vi "MotionCapture0429.vi"() -> ()   [LabVIEW 2020]
uses:
  <vilib>/Math Plots/3D Math Plots/3D Scatter/3D Scatter XCtrl/3D Scatter.xctl
  <vilib>/Math Plots/3D Math Plots/3D Scatter/3D Scatter Datatype/3D Scatter Datatype.lvclass
  <vilib>/imath/engines/lvmath2/RunTimeEngine/IndexRead/NIMS V(S).vi
  <instcachedir>/0/NIMS V(S)_0488751826AF41519A22953C041130DC.lvgen/NIMS V(S)_0488751826AF41519A22953C041130DC_000.vi
  <vilib>/imathl/engines/lvmath/Functions/Error Handling/Create Error.vi
  <vilib>/imath/engines/lvmath2/RunTimeEngine/BuiltInFunctions/norm/NIMS_norm(GV,DBL).vi
  <instcachedir>/0/NIMS_norm(GV,DBL)_118B4CCB667A4D7498CD7C123070720C.lvgen/NIMS_norm(GV,DBL)_118B4CCB667A4D7498CD7C123070720C_000.vi
  <vilib>/imath/engines/lvmath2/RunTimeEngine/BuiltInFunctions/dot/NIMS_dot(GV,GV).vi
  <instcachedir>/0/NIMS_dot(GV,GV)_B9FAA411F4494E9B94D442721014A3FA.lvgen/NIMS_dot(GV,GV)_B9FAA411F4494E9B94D442721014A3FA_000.vi
  <vilib>/imath/engines/lvmath2/RunTimeEngine/ErrorHandling/NIMS_Create Error From Enums.vi
  <vilib>/imath/engines/lvmath2/RunTimeEngine/BuiltInFunctions/atan2/NIMS_atan2.vi
  <instcachedir>/0/NIMS_atan2_A91AA4A7D42247EDBE8F76DB99AF04A4.lvgen/NIMS_atan2_A91AA4A7D42247EDBE8F76DB99AF04A4_000.vi
  <vilib>/imath/engines/lvmath2/RunTimeEngine/BuiltInFunctions/sin/NIMS_sin(C).vi
  <instcachedir>/0/NIMS_sin(C)_5976CC71585441B3B5B50155927B54AC.lvgen/NIMS_sin(C)_5976CC71585441B3B5B50155927B54AC_001.vi
  <vilib>/imath/engines/lvmath2/RunTimeEngine/NodeEndStatement/NIMS_NodeEndStatement_Output.vi
  <instcachedir>/0/NIMS_NodeEndStatement_Output_53EC0D466D134D7ABD903AC30B43404B.lvgen/NIMS_NodeEndStatement_Output_53EC0D466D134D7ABD903AC30B43404B_001.vi
  <instcachedir>/0/NIMS_NodeEndStatement_Output_53EC0D466D134D7ABD903AC30B43404B.lvgen/NIMS_NodeEndStatement_Output_53EC0D466D134D7ABD903AC30B43404B_009.vi
  <vilib>/imath/engines/lvmath2/RunTimeEngine/ErrorHandling/NIMS_Finalize Error.vi
  <vilib>/Math Plots/3D Math Plots/3D Scatter/3D Scatter Datatype/Public/Plot Helper (Vector).vi
panel:
  out "3D Scatter":refnum<class "3D Plot Datatype.lvclass">[](xcontrol) caption="Endpoint Trajectory"
  in  "采集开关":bool=TRUE
  in  "BodyID":dbl=14.0
  out "CMTrackData":T1={"BodyID"=5, "timecode"=1444098, "T"=[230.07000732421875, 348.40191650390625, -6.298731803894043], [0.322020434693915, 0.3319248787086055, 0.6304688324459874, -0.623408185579892]}
  in  "BodyID 2":dbl=1550.0
  out "CMTrackData 2":T1={"BodyID"=1550, "timecode"=1444098, "T"=[269.41546630859375, 348.2109680175781, 32.023807525634766], [0.0, 1.0, 0.0, 0.0]}
  in  "BodyID 3":dbl=1551.0
  out "CMTrackData 3":T1={"BodyID"=1551, "timecode"=1376028, "T"=[269.479248046875, 346.3133850097656, -49.665985107421875], [0.0, 1.0, 0.0, 0.0]}
  in  "BodyID 4":dbl=1552.0
  out "CMTrackData 4":T1={"BodyID"=1552, "timecode"=1444098, "T"=[187.96241760253906, 347.5824279785156, -41.51162338256836], [0.0, 1.0, 0.0, 0.0]}
  in  "BodyID 5":dbl=16.0
  out "CMTrackData 5":T1={"BodyID"=4, "timecode"=1444098, "T"=[-277.2441711425781, 137.65509033203125, -26.613216400146484], [0.9980943925853861, 0.015375121692000475, 0.004095479898044867, -0.05961892457072499]}
  in  "BodyID 6":dbl=1500.0
  out "CMTrackData 6":T1={"BodyID"=1500, "timecode"=1444098, "T"=[-291.25531005859375, 185.45095825195312, -25.36912727355957], [0.0, 1.0, 0.0, 0.0]}
  in  "BodyID 7":dbl=1501.0
  out "CMTrackData 7":T1={"BodyID"=1501, "timecode"=1444098, "T"=[-309.5177307128906, 100.24006652832031, -25.89438247680664], [0.0, 1.0, 0.0, 0.0]}
  in  "BodyID 8":dbl=1502.0
  out "CMTrackData 8":T1={"BodyID"=1502, "timecode"=1444098, "T"=[-324.59747314453125, 148.97030639648438, -25.411792755126953], [0.0, 1.0, 0.0, 0.0]}
  out "qRotated 2":dbl[](array[numeric])=[0.0, 303.37976210106535, -404.89104773175404, 214.9849718318804]
  in  "错误输入":errorcluster
  out "错误输出":errorcluster
  out "l":cdb=334.3417003066229-0.0i
  out "theta":cdb=1.5549921643579725-0.0i
  out "phi":dbl=-0.9277514353888752
  out "Endpoint XYZ":cluster{dbl, dbl, dbl}(graph)={303.37976210106535, -404.89104773175404, 214.9849718318804}
  out "Length":dbl(graph)=334.3417003066229
  out "Theta":dbl(graph)=1.5549921643579725
  out "Phi":dbl(graph)=-0.9277514353888752
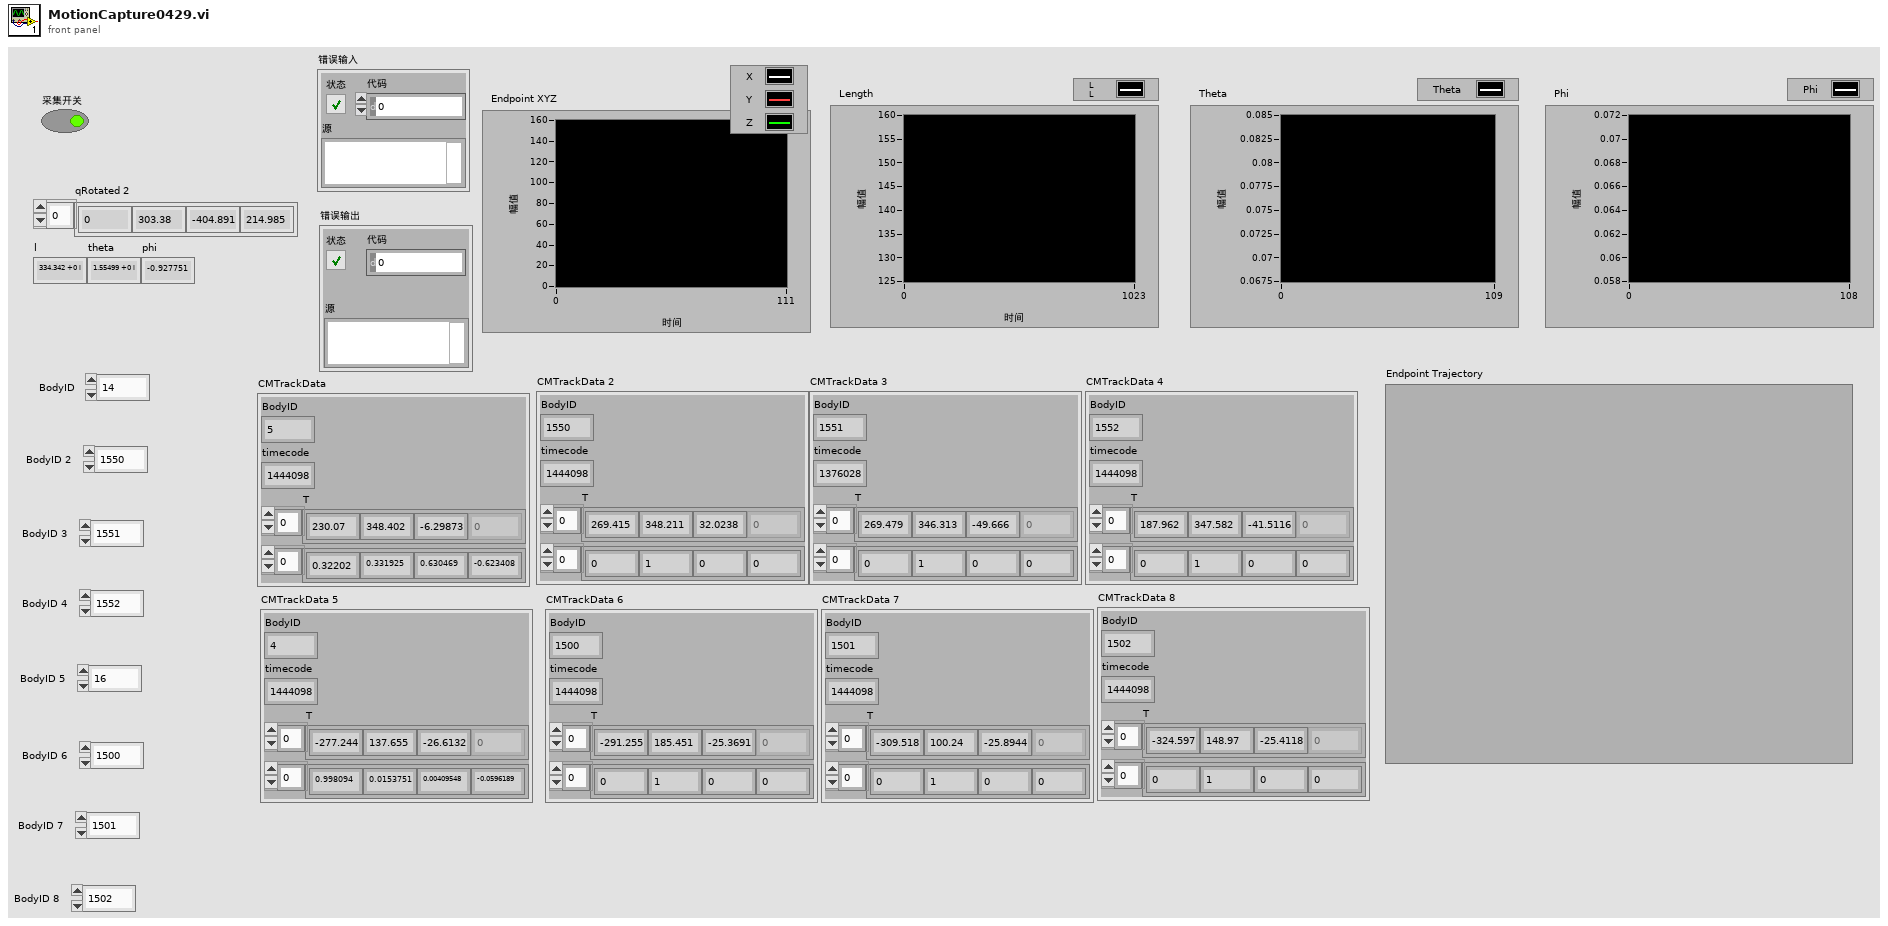
[diagram p1: front panel]
types:
  T1 = cluster{"BodyID":i32, "timecode":i32, "T":dbl[], dbl[]}
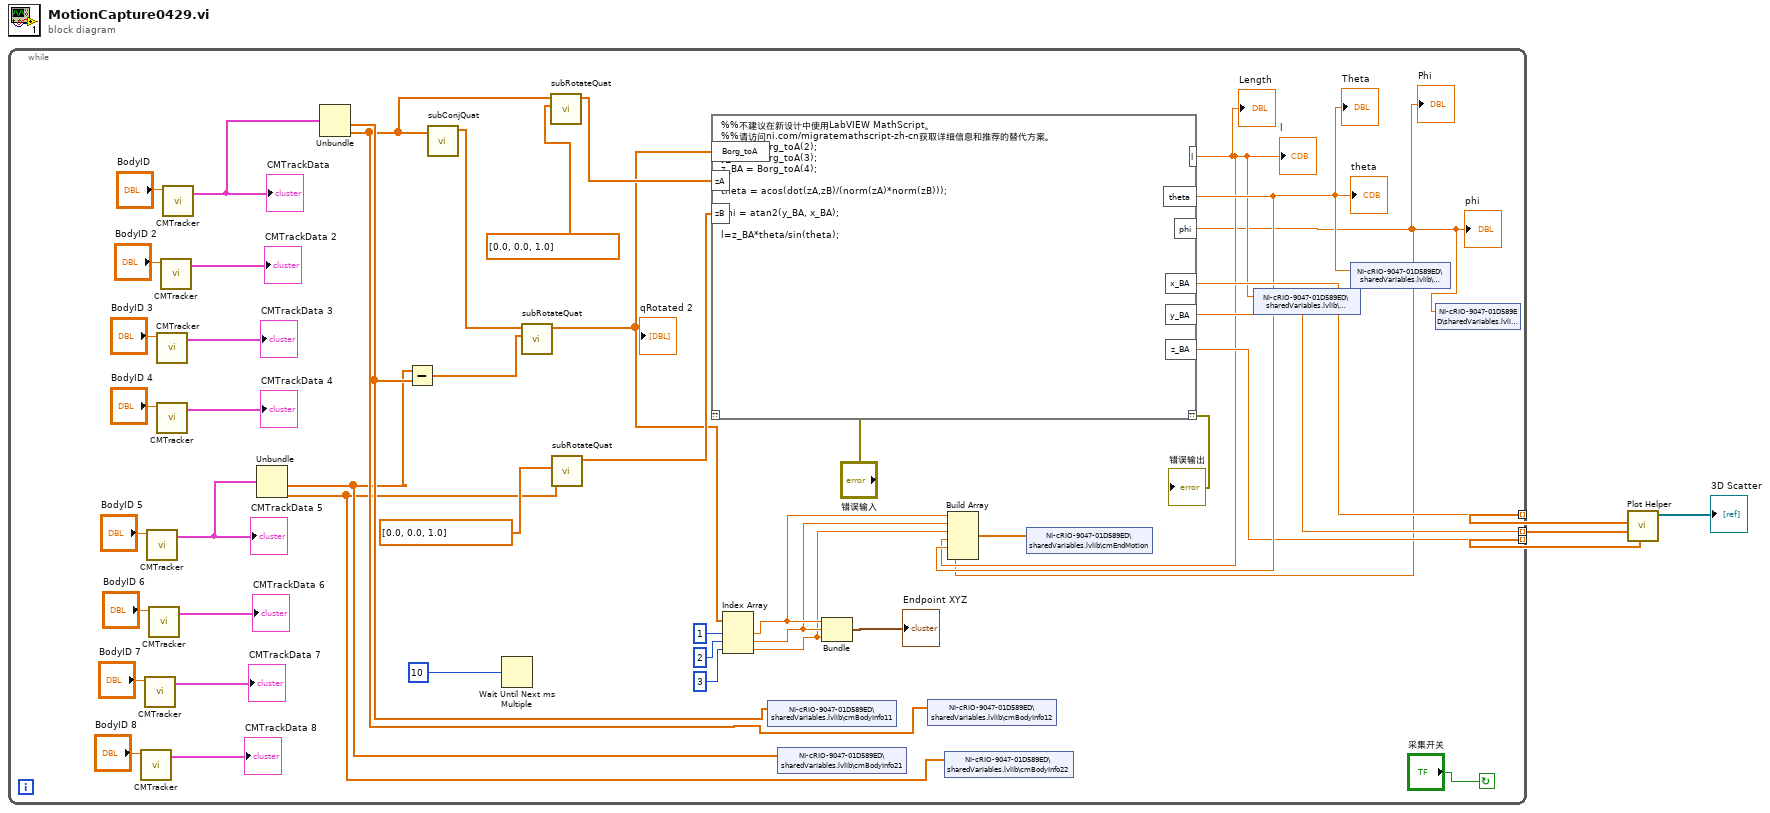
[diagram p0: block diagram]
diagram:
  n1 = while {
    tunnel: [w24] -> w3 mode=indexing
    tunnel: [w23] -> w2 mode=indexing
    tunnel: [w12] -> w1 mode=indexing
    stop <- "采集开关" continue-if-true
    n2 = call "CMTracker.vi"("BodyID"="BodyID 8") -> ("CMTrackData"=→"CMTrackData 8":T1)  [unwired: 10 in]
    n3 = call "CMTracker.vi"("BodyID"="BodyID 7") -> ("CMTrackData"=→"CMTrackData 7":T1)  [unwired: 10 in]
    n4 = call "CMTracker.vi"("BodyID"="BodyID 5") -> ("CMTrackData"=w33:T1)  [unwired: 10 in]
    "CMTrackData 5" <- w33
    n5 = call "CMTracker.vi"("BodyID"="BodyID 6") -> ("CMTrackData"=→"CMTrackData 6":T1)  [unwired: 10 in]
    n6 = call "CMTracker.vi"("BodyID"="BodyID 3") -> ("CMTrackData"=→"CMTrackData 3":T1)  [unwired: 10 in]
    n7 = call "CMTracker.vi"("BodyID"="BodyID 4") -> ("CMTrackData"=→"CMTrackData 4":T1)  [unwired: 10 in]
    n8 = call "CMTracker.vi"("BodyID"="BodyID 2") -> ("CMTrackData"=→"CMTrackData 2":T1)  [unwired: 10 in]
    n9 = call "CMTracker.vi"("BodyID"="BodyID") -> ("CMTrackData"=w34:T1)  [unwired: 10 in]
    "CMTrackData" <- w34
    n10 = Unbundle(w33) -> ("T"=w6:dbl[], w5:dbl[])  [unwired: 2 out]
    n11 = Unbundle(w34) -> ("T"=w8:dbl[], w7:dbl[])  [unwired: 2 out]
    n12 = Subtract(x=w6, y=w8) -> (x-y=w32:dbl[])
    n13 = call "subConjQuat.vi"("q"=w7) -> ("qConj"=w25:dbl[])  [unwired: 10 in]
    n14 = Wait Until Next ms Multiple(millisecond multiple=10) -> ()  [unwired: 1 out]
    n15 = call "subRotateQuat.vi"("dotToTotate"=w32, "q"=w25) -> ("qRotated"=w18:dbl[])  [unwired: 9 in]
    "qRotated 2" <- w18
    n16 = call "subRotateQuat.vi"("dotToTotate"=dbl[] [0.0, 0.0, 1.0], "q"=w7) -> ("qRotated"=w28:dbl[])  [unwired: 9 in]
    n17 = call "subRotateQuat.vi"("dotToTotate"=dbl[] [0.0, 0.0, 1.0], "q"=w5) -> ("qRotated"=w30:dbl[])  [unwired: 9 in]
    n18 = mathscript code="%%不建议在新设计中使用LabVIEW MathScript。\n%%请访问ni.com/migratemathscript-zh-cn获取详细信息和推荐的替代方案。\nx_BA = Borg_toA(2);\ny_BA = Borg_toA(3);\nz_BA = Borg_toA(4);\n\ntheta = acos(dot(zA,zB)/(norm(zA)*norm(zB)));\n\nphi = atan2(y_BA, x_BA);\n\nl=z_BA*theta/sin(theta);"("??"="错误输入", "Borg_toA"=w18, "zA"=w28, "zB"=w30) -> ("??"=→"错误输出":errorcluster, "l"=w10:cdb, "theta"=w13:cdb, "phi"=w9:dbl, "x_BA"=w24:dbl, "y_BA"=w23:dbl, "z_BA"=w12:dbl)
    "l" <- w10
    "theta" <- w13
    "phi" <- w9
    "Length" <- w10
    "Theta" <- w13
    "Phi" <- w9
    n19 = Index Array(array=w18, index #1=1, index #2=2, index #3=3) -> (element #1=w17:dbl, element #2=w16:dbl, element #3=w11:dbl)
    n20 = shared-variable "NI-cRIO-9047-01D589ED\\sharedVariables.lvlib\\cmBodyInfo11"(w8) -> ()  [unwired: 1 in, 1 out]
    n21 = shared-variable "NI-cRIO-9047-01D589ED\\sharedVariables.lvlib\\cmBodyInfo21"(w6) -> ()  [unwired: 1 in, 1 out]
    n22 = Bundle("数值"=w17, "数值"=w16, "数值"=w11) -> (→"Endpoint XYZ":cluster{"数值":dbl, "数值":dbl, "数值":dbl})  [unwired: 1 in]
    n23 = shared-variable "NI-cRIO-9047-01D589ED\\sharedVariables.lvlib\\cmBodyInfo12"(w7) -> ()  [unwired: 1 in, 1 out]
    n24 = shared-variable "NI-cRIO-9047-01D589ED\\sharedVariables.lvlib\\cmBodyInfo22"(w5) -> ()  [unwired: 1 in, 1 out]
    n25 = Build Array(w17, w16, w11, w10, w13, w9) -> (w15:cdb[])
    n26 = shared-variable "NI-cRIO-9047-01D589ED\\sharedVariables.lvlib\\cmEndMotion"(w15) -> ()  [unwired: 1 in, 1 out]
    n27 = shared-variable "NI-cRIO-9047-01D589ED\\sharedVariables.lvlib\\armLength"(w10) -> ()  [unwired: 1 in, 1 out]
    n28 = shared-variable "NI-cRIO-9047-01D589ED\\sharedVariables.lvlib\\armTheta"(w13) -> ()  [unwired: 1 in, 1 out]
    n29 = shared-variable "NI-cRIO-9047-01D589ED\\sharedVariables.lvlib\\armPhi"(w9) -> ()  [unwired: 1 in, 1 out]
  }
  n30 = call-poly <vilib>:"Plot Helper.vi"("z vector"=w1, "y vector"=w2, "x vector"=w3) -> ("3D Plot lvclass Array out"=→"3D Scatter":refnum<class "3D Plot Datatype.lvclass">[])  [unwired: 3 in, 5 out]
